vi "CSM_adm_0@8.vi"(4 "err in":errorcluster, 5 "q":dbl, 6 "Cc":dbl, 7 "Qa":dbl) -> (0 "err out":errorcluster, 3 "Cadm":dbl)   [LabVIEW 2010, in "lv_07.lvlib"]
doc: "Calcul le coût administratif (gestion des commandes) en fonction de Qa et Cc et de la variable q : Qté commandée à chaque commande. Pour cette quantité q, Nc=Qa/q est donc le nombre de commandes passées à l'année.\nq doit être >0"
uses:
  lv_07.lvlib
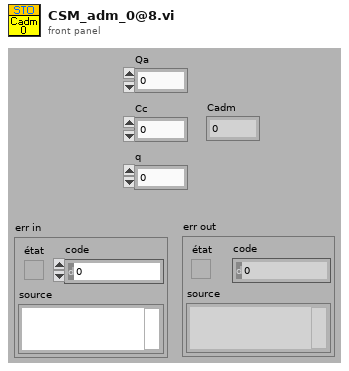
[diagram p1: front panel]
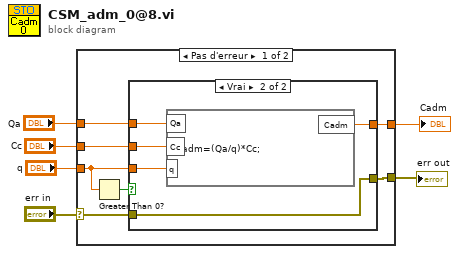
[diagram p0: block diagram]
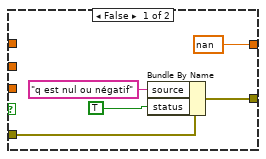
[diagram p2: hidden frame]
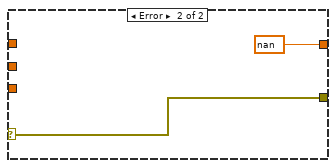
[diagram p3: hidden frame]
diagram:
  n1 = case shown="Pas d'erreur" "err in" {
    selector: "err in" -> [w8 w25]
    tunnel: [w13 nan ("Cadm")] -> w6
    tunnel: "Qa" -> [w12 _]
    tunnel: "Cc" -> [w11 _]
    tunnel: "q" -> [w9 _]
    tunnel: [w7 w25] -> w1
    frame No Error {
      n2 = Greater Than 0?(x=w9) -> (x > 0?=w10:bool)
      n3 = case shown="Vrai" w10 {
        tunnel: [nan ("Cadm") w23] -> w13
        tunnel: w12 -> [_ w22]
        tunnel: w11 -> [_ w21]
        tunnel: w9 -> [_ w20]
        tunnel: w8 -> [w17 w19]
        tunnel: [w14 w19] -> w7
        frame False {
          n4 = Bundle By Name(cluster=w17, "source"="q est nul ou négatif", "status"=TRUE) -> (w14:errorcluster)
        }
        frame True {
          n5 = formula code="Cadm=(Qa/q)*Cc;"("Qa"=w22, "Cc"=w21, "q"=w20) -> ("Cadm"=w23:dbl)
        }
      }
    }
    frame Error {
    }
  }
  "Cadm" <- w6
  "err out" <- w1
